vi "JKISM++ Unregistrer Status Change.vi"(0 "JKISM Name":string, 5 "Source JKISM Name":string="*", 7 "Status":string, 11 "Error in":errorcluster caption="Error in (no error)") -> (4 "JKISM Name(dup)":string, 15 "Error out":errorcluster)   [LabVIEW 2014, in "JKI-State-Machine-Plus.lvlib"]
uses:
  JKI-State-Machine-Plus.lvlib
  _Support/FGV-BroadcastRegistry/Oper-BroadcastRegistry.ctl
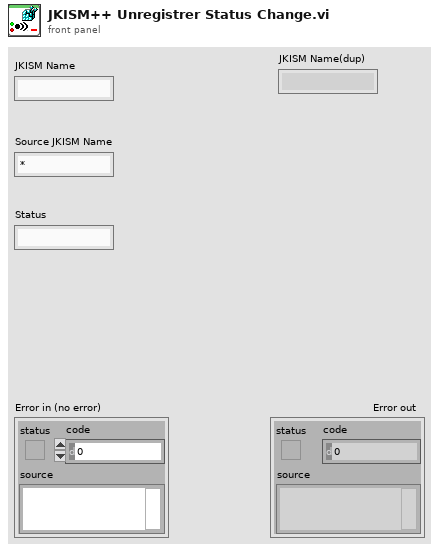
[diagram p1: front panel]
types:
  T1 = typedef "JKI-State-Machine-Plus.lvlib/Oper-BroadcastRegistry.ctl" = enum16{"Delete Source Module", "Delete Dest Module", "Remove Module", "Register", "Unregister", "Check"}
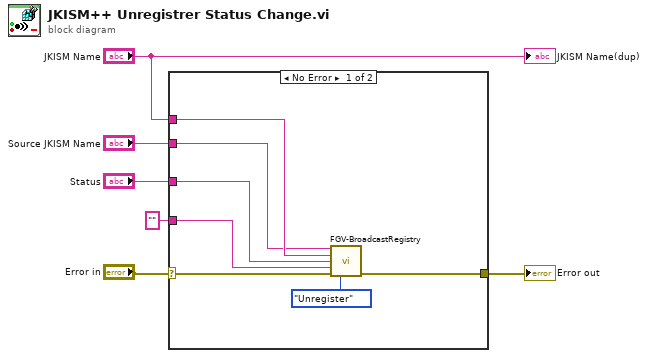
[diagram p0: block diagram]
diagram:
  n1 = case shown="No Error" "Error in" {
    selector: "Error in" -> [w12 w14]
    tunnel: [w11 w14] -> w5
    tunnel: "" ("ActingMsg") -> [w10 _]
    tunnel: "Status" -> [w9 _]
    tunnel: "Source JKISM Name" -> [w7 _]
    tunnel: "JKISM Name" -> [w8 _]
    frame No Error {
      n2 = call "FGV-BroadcastRegistry.vi"("Source"=w7, "Dest"=w8, "Message"=w9, "ActingMsg In"=w10, "Error in"=w12, "Operation"=Oper-BroadcastRegistry."Unregister") -> ("Error out"=w11:errorcluster)  [unwired: 7 in, 2 out]
    }
    frame Error {
    }
  }
  "Error out" <- w5
  "JKISM Name(dup)" <- "JKISM Name"
